vi "Curtin_ReadColor.vi"(3 "color file name":string) -> (0 "Success?":bool, 1 "Colors":u32[](array[numeric]))   [LabVIEW 2022 SP3]
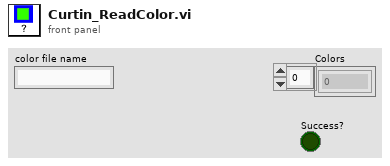
[diagram p1: front panel]
types:
  T1 = enum16{"big-endian, network order", "native, host order", "little-endian"}
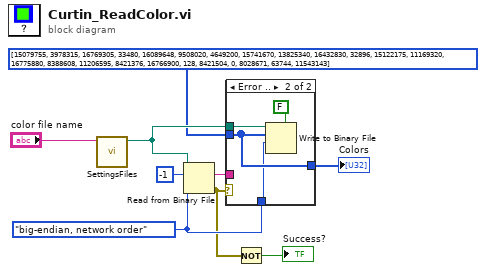
[diagram p0: block diagram]
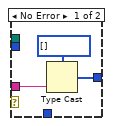
[diagram p2: hidden frame]
diagram:
  w3 = T1."big-endian, network order" ("byte order (0:big-endian, network order)")
  n1 = call "SettingsFiles.vi"("settings file name"="color file name") -> ("file path"=w9:path)  [unwired: 9 in, 1 out]
  n2 = Read from Binary File(9:w3, 10:-1 ("count (1)"), 11:w9) -> (0:w2:errorcluster, 2:w4:string)  [unwired: 3 in, 2 out]
  n3 = case shown="Error .." w2 {
    tunnel: w4 -> [w11 _]
    tunnel: [w10 w15] -> w6
    tunnel: u32[] [15079755, 3978315, 16769305, 33480, 16089648, 9508020, 4649200, 15741670, 13825340, 16432830, 32896, 15122175, 11169320, 16775880, 8388608, 11206595, 8421376, 16766900, 128, 8421504, 0, 8028671, 63744, 11543143] ("Colors") -> [_ w15]
    tunnel: w9 -> [_ w14]
    tunnel: w3 -> [_ w13]
    frame No Error {
      n4 = Type Cast(type=u32[] [] ("Color"), x=w11) -> (*(type *) &x=w10:u32[])
    }
    frame Error {
      n5 = Write to Binary File(file (use dialog)=w14, data=w15, 5:FALSE ("prepend array or string size? (T)"), 9:w13) -> ()  [unwired: 2 in, 3 out]
    }
  }
  "Colors" <- w6
  n6 = Not(x=w2) -> (.not. x?=→"Success?":bool)
